vi "Resolve Flow Directive.vi"(4 "Remaining in":string, 6 "Directive":string, 7 "Folder":path, 8 "error in (no error)":errorcluster, 9 "Locals in":refnum<class "Value Tree.lvclass">, 10 "Value Name":string, 11 "BasicTemplater in":refnum<class "BasicTemplater.lvclass">) -> (0 "error out":errorcluster, 1 "Remaining":string, 2 "Value":refnum<class "Value Tree.lvclass">, 3 "BasicTemplater out":refnum<class "BasicTemplater.lvclass">)   [LabVIEW 2020, in "HTTP Server.lvlib" / "BasicTemplater.lvclass"]
uses:
  BasicTemplater.lvclass
  Value Tree/Value Tree.lvclass
  BasicTemplater.lvclass/BasicTemplater.ctl
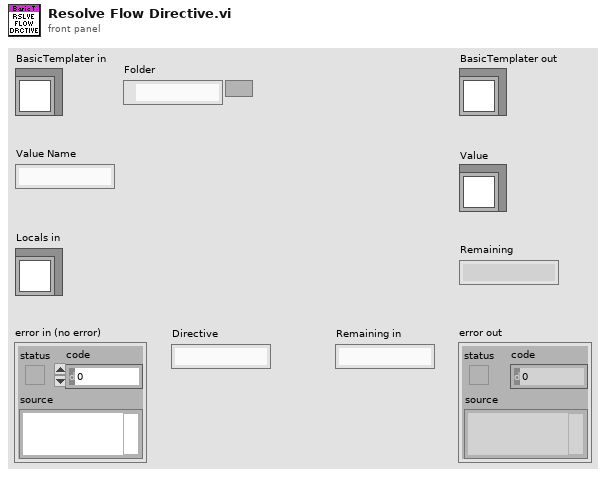
[diagram p1: front panel]
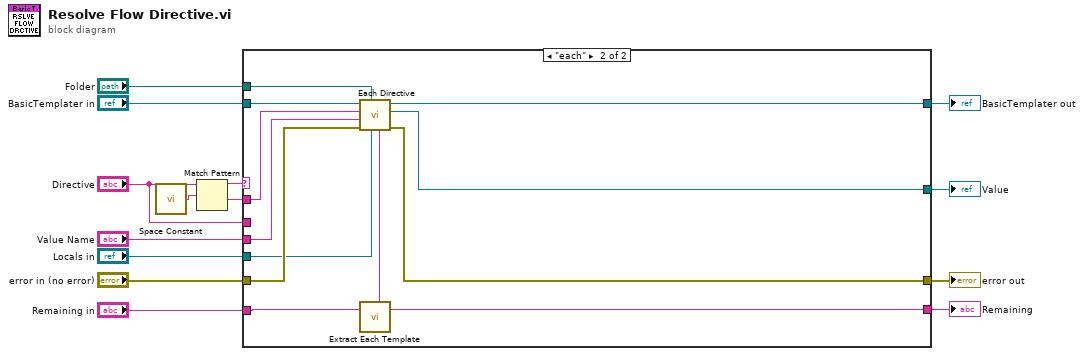
[diagram p0: block diagram]
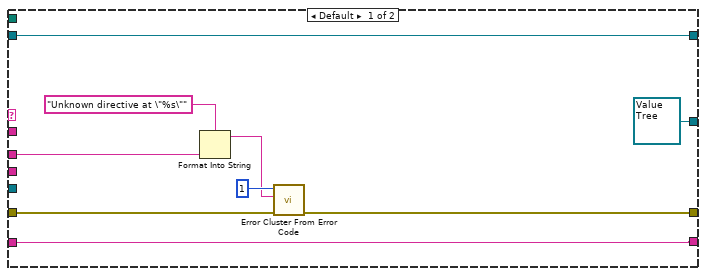
[diagram p2: hidden frame]
diagram:
  n1 = call <vilib>:"Space Constant.vi"() -> ("String"=w14:string)
  n2 = Match Pattern(string="Directive", regular expression=w14) -> (before substring=w13:string, after substring=w12:string)  [unwired: 1 in, 2 out]
  n3 = case shown="\"each\"" w13 {
    tunnel: w12 -> [_ w29]
    tunnel: "Locals in" -> [_ w27]
    tunnel: "BasicTemplater in" -> [w23 w34]
    tunnel: "Folder" -> [_ w33]
    tunnel: [w21 w32] -> w4
    tunnel: [w23 w31] -> w9
    tunnel: [refnum<class "Value Tree.lvclass"> refnum ("Value") w30] -> w8
    tunnel: "Directive" -> [w17 _]
    tunnel: "error in (no error)" -> [w16 w35]
    tunnel: "Value Name" -> [_ w28]
    tunnel: "Remaining in" -> [w15 w26]
    tunnel: [w15 w24] -> w1
    frame Default {
      n4 = Format Into String(format string="Unknown directive at \"%s\"", w17) -> (resulting string=w18:string)  [unwired: 2 in, 1 out]
      n5 = call <vilib>:"Error Cluster From Error Code.vi"("error in (no error)"=w16, "error message (\"\")"=w18, "error code (0)"=1) -> ("error out"=w21:errorcluster)  [unwired: 6 in]
    }
    frame "each" {
      n6 = call "Extract Each Template.vi"("Remaining in"=w26) -> ("Template"=w25:string, "Remaining"=w24:string)  [unwired: 5 in]
      n7 = call "Each Directive.vi"("Template"=w25, "Locals"=w27, "Folder"=w33, "error in (no error)"=w35, "Value Name"=w28, "Directive"=w29, "BasicTemplater in"=w34) -> ("error out"=w32:errorcluster, "Value"=w30:refnum<class "Value Tree.lvclass">, "BasicTemplater out"=w31:refnum<class "BasicTemplater.lvclass">)  [unwired: 2 in]
    }
  }
  "error out" <- w4
  "BasicTemplater out" <- w9
  "Value" <- w8
  "Remaining" <- w1
